vi "가운데로(subVI).vi"(8 "에러 입력(에러 없음)":errorcluster, 11 "VI 입력":refnum<vi>) -> (0 "에러 출력":errorcluster, 3 "VI 출력":refnum<vi>)   [LabVIEW 2014]
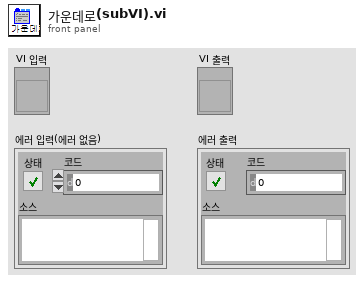
[diagram p1: front panel]
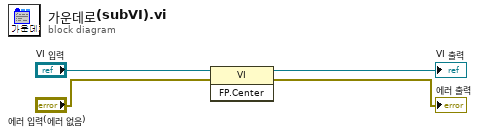
[diagram p0: block diagram]
diagram:
  n1 = invoke class="VI" method="FP.Center"(reference="VI 입력", error in="에러 입력(에러 없음)") -> (reference out=→"VI 출력":refnum<vi>, error out=→"에러 출력":errorcluster)  [unwired: 1 in, 1 out]
